vi "MOKE-5-23-22.vi"() -> ()   [LabVIEW 2021]
uses:
  <vilib>/Analysis/NI_AALBase.lvlib
  <vilib>/Analysis/baseanly.llb/Mean (DBL).vi
  <vilib>/Analysis/Matrix/Datatypes/RealMatrix.ctl
  <vilib>/Analysis/Matrix/NI_Matrix.lvlib
panel:
  out "photodiode live avg graph (plots every average, need to update)":cluster{"Y":dbl[], "Y":dbl[]}[](graph)
  out "photodiode final avg graph":cluster{"Y":dbl[], "Y":dbl[]}[](graph)
  out "avgs  (missing last two values but that's ok ig)":dbl[](array[numeric])
  out "avg":dbl
  out "col_arr":dbl[][](array[numeric])
  in  "blank":dbl[](array[numeric])
  out "y_mat":T1
  in  "stop":bool
  in  "Total Loops":dbl
  out "Current Loop":i32
  in  "Time / Step":i64
  in  "Number of Samples":i32=100
  out "Graph For Photodiode":cluster{"Y":dbl[], "Y":dbl[]}[](graph)
  out "Photodiode Level":dbl
  out "Current Voltage":dbl
  in  "Scans From 0 to Max Voltage":i32
  in  "Voltage":dbl
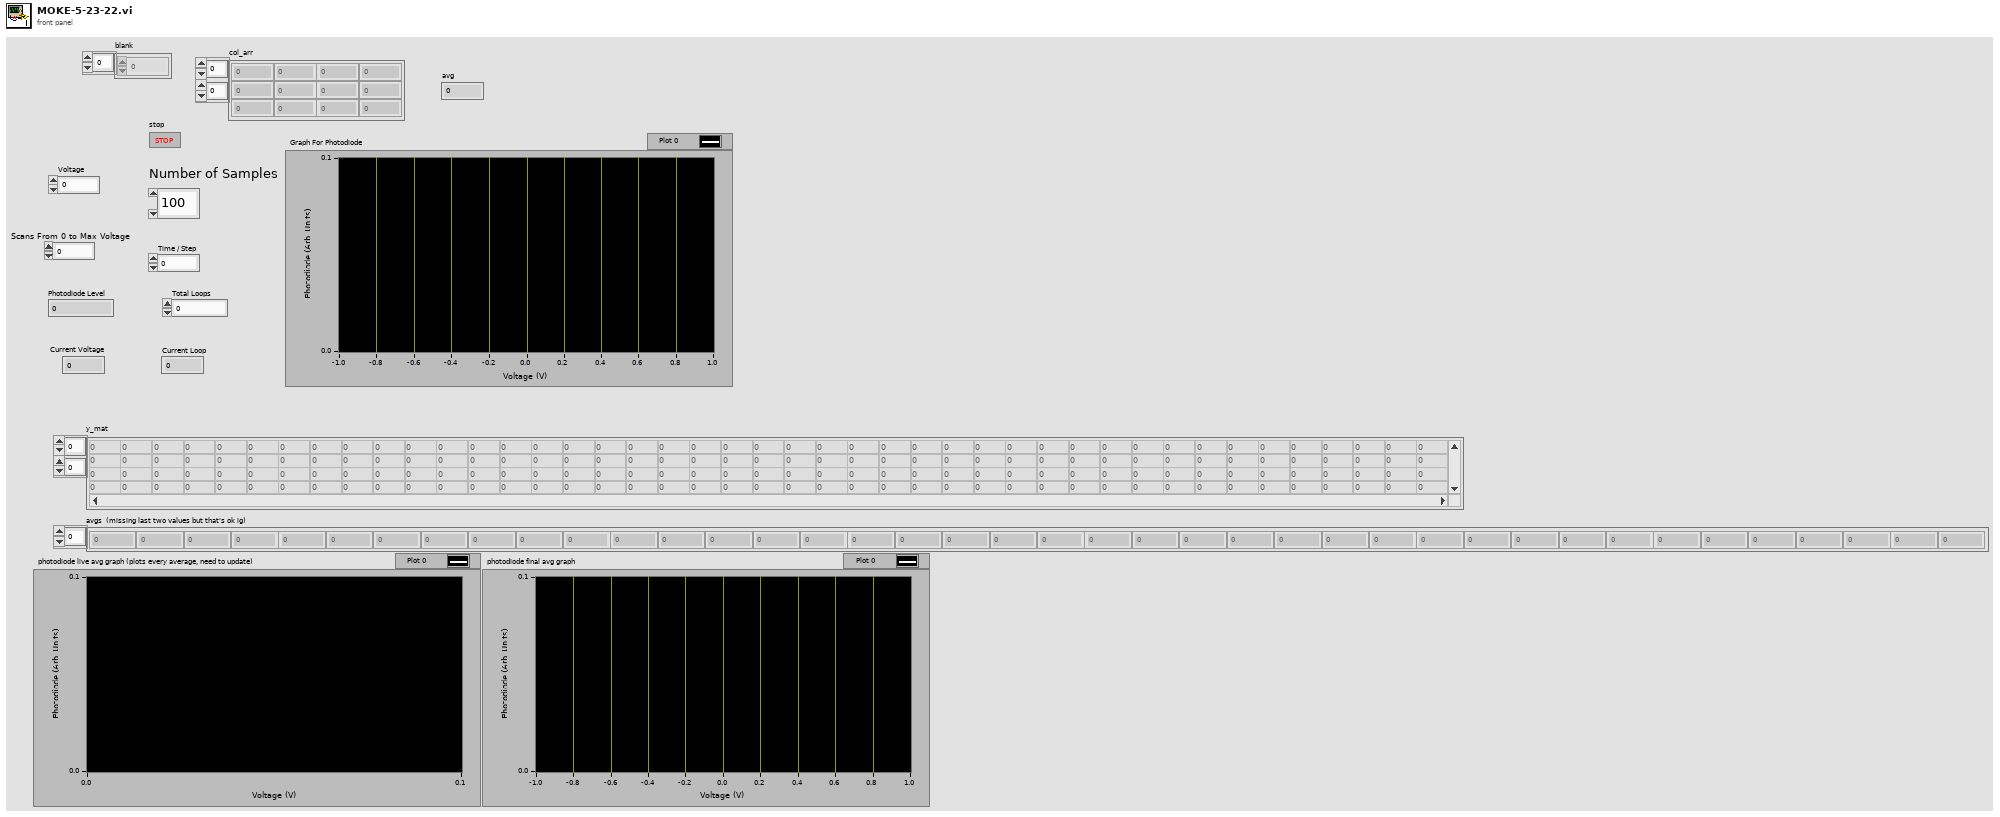
[diagram p1: front panel]
types:
  T1 = typedef "NI_Matrix.lvlib/RealMatrix.ctl" = dbl[][]
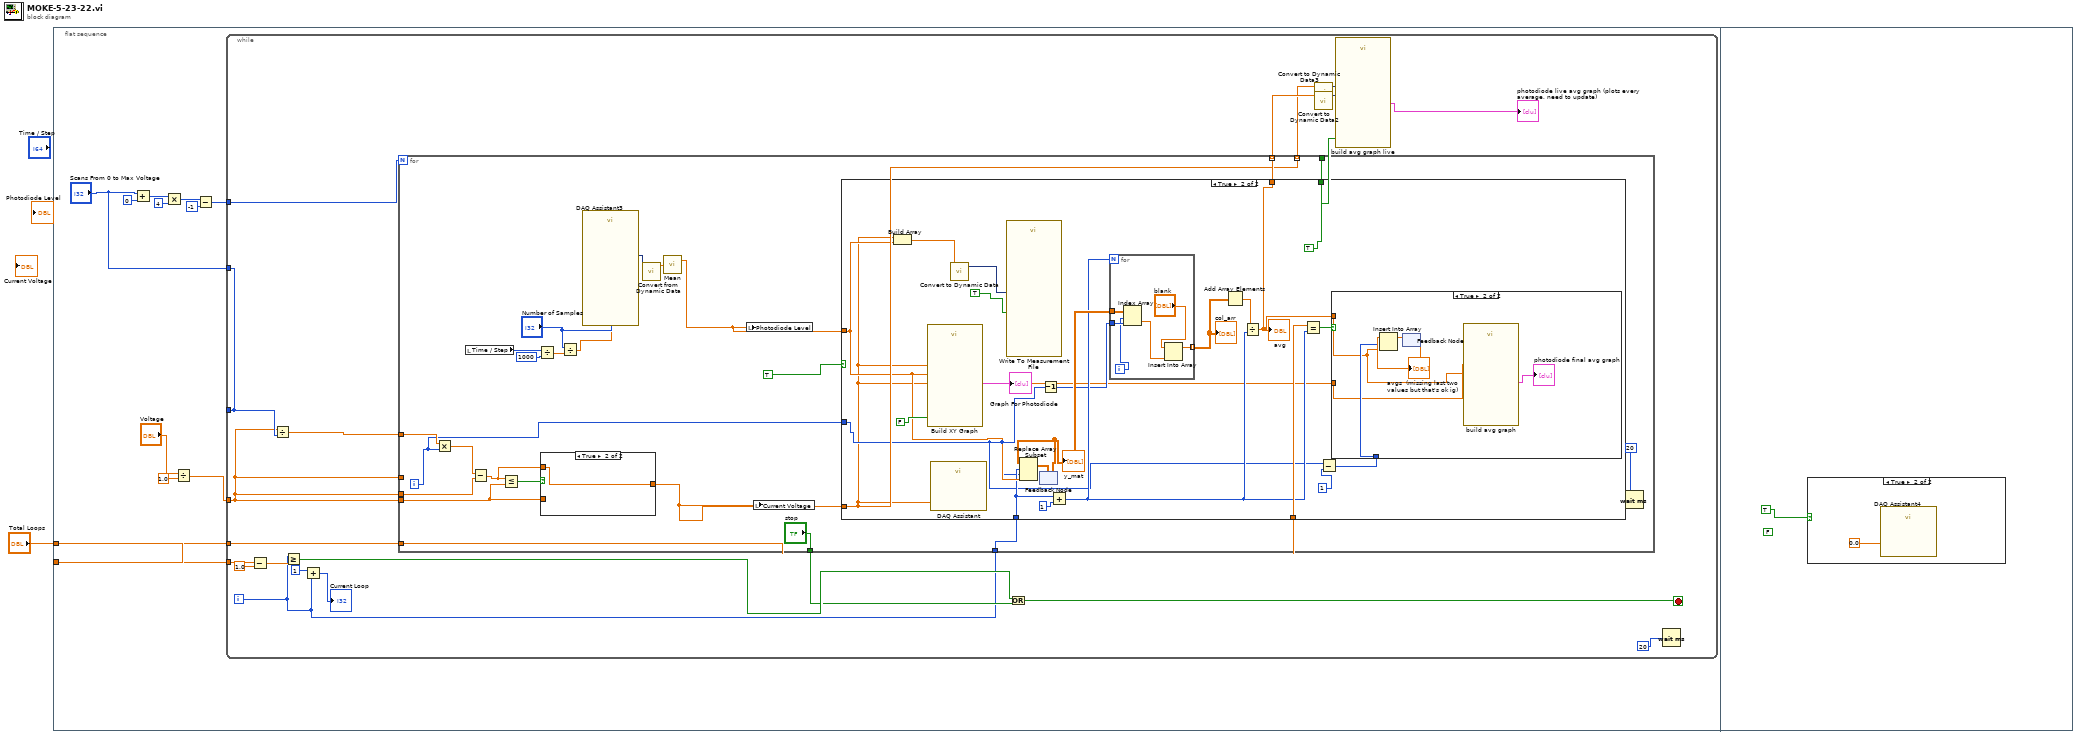
[diagram p0: block diagram]
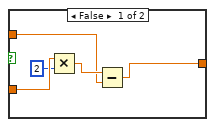
[diagram p2: hidden frame]
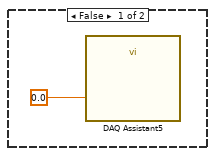
[diagram p5: hidden frame]
diagram:
  n1 = flat-sequence {
    tunnel: "Total Loops" -> [w6]
    tunnel: "Total Loops" -> [w2]
    frame #0 {
      n2 = Add(x="Scans From 0 to Max Voltage", y=0) -> (x+y=w12:i32)
      n3 = Multiply(x=w12, y=4) -> (x*y=w13:i32)
      n4 = Divide(x="Voltage", y=1.0) -> (x/y=w3:dbl)
      n5 = Subtract(x=w13, y=-1) -> (x-y=w8:i32)
      n6 = while {
        tunnel: w6 -> [w33]
        tunnel: [w24] -> _
        tunnel: w8 -> [w25]
        tunnel: "Scans From 0 to Max Voltage" -> [w24]
        tunnel: w3 -> [w23]
        tunnel: w2 -> [w20]
        i -> [w21]
        stop <- w27 stop-if-true
        n7 = Subtract(x=w33, y=1.0) -> (x-y=w32:dbl)
        n8 = Divide(x=w23, y=w24) -> (x/y=w34:dbl)
        n9 = Greater Or Equal?(x=w21, y=w32) -> (x >= y?=w28:bool)
        n10 = Add(x=1, y=w21) -> (x+y=→"Current Loop":i32)
        n11 = for {
          N: w25 -> [_]
          tunnel: w34 -> [w58]
          tunnel: w23 -> [_]
          tunnel: w23 -> [w55]
          tunnel: w23 -> [w51]
          tunnel: ["stop"] -> w26
          tunnel: w21 -> [w39]
          tunnel: w20 -> [w38]
          tunnel: [w37] -> w19
          tunnel: [w36] -> w18 mode=indexing
          tunnel: [w35] -> w17 mode=indexing
          i -> [w40]
          n12 = Multiply(x=w58, y=w40) -> (x*y=w56:dbl)
          n13 = local read "Time / Step"() -> (w47:i64)
          n14 = Subtract(x=w56, y=w55) -> (x-y=w53:dbl)
          n15 = Less Or Equal?(x=w53, y=w51) -> (x <= y?=w54:bool)
          n16 = Divide(x=w47, y=i64 1000) -> (x/y=w48:dbl)
          n17 = case shown="True" w54 {
            tunnel: w53 -> [w60 w64]
            tunnel: [w59 w64] -> w52
            tunnel: w51 -> [w63 _]
            frame False {
              n18 = Multiply(x=w63, y=2) -> (x*y=w61:dbl)
              n19 = Subtract(x=w61, y=w60) -> (x-y=w59:dbl)
            }
            frame True {
            }
          }
          n20 = Divide(x="Number of Samples", y=w48) -> (x/y=w49:dbl)
          n21 = call "DAQ Assistant3"("rate"=w49, "number of samples"="Number of Samples") -> ("data"=w45:dynamicdata)  [unwired: 4 in, 13 out]
          n22 = call "Convert from Dynamic Data"("Dynamic Data Type"=w45) -> ("Array"=w44:dbl[])  [unwired: 3 in]
          n23 = call-poly <vilib>:"Mean.vi"("X"=w44) -> ("mean"=w43:dbl)  [unwired: 1 out]
          n24 = local write "Photodiode Level"(w43) -> ()
          n25 = local write "Current Voltage"(w52) -> ()
          n26 = case shown="True" TRUE {
            tunnel: w52 -> [_ w65]
            tunnel: w43 -> [_ w81]
            tunnel: w40 -> [_ w69]
            tunnel: w39 -> [_ w76]
            tunnel: w38 -> [_ w75]
            tunnel: [_ TRUE] -> w37
            tunnel: [_ w66] -> w36
            tunnel: [_ w65] -> w35
            frame False {
            }
            frame True {
              n27 = Build Array(w65, w81) -> (w84:dbl[])
              n28 = call "Build XY Graph"("Reset"=FALSE, "Y Input"=w81, "X Input"=w65) -> ("XY Graph"=→"Graph For Photodiode":cluster{"X":dbl[], "Y":dbl[]}[])  [unwired: 7 in, 1 out]
              n29 = call "DAQ Assistant"("data"=w65) -> ()  [unwired: 17 in, 2 out]
              n30 = call "Convert to Dynamic Data"("Array"=w84) -> ("Dynamic Data Type"=w82:dynamicdata)  [unwired: 3 in]
              n31 = call "Write To Measurement File"("Signals"=w82, "Enable"=TRUE) -> ()  [unwired: 15 in, 3 out]
              n32 = feedback #1() -> (w79:T1)  [unwired: 1 in]
              "y_mat" <- w79
              n33 = Replace Array Subset(array=w79, new element=w81, index (row)=w76, index (col)=w69) -> (w80:T1)
              n34 = feedback-in #1(w80) -> ()
              n35 = Decrement(x=w69) -> (x-1=w70:i32)
              n36 = Add(x=w76, y=1) -> (x+y=w71:i32)
              n37 = for {
                N: w71 -> [_]
                tunnel: w79 -> [w98]
                tunnel: w70 -> [w94]
                tunnel: [w95] -> w68 mode=indexing
                i -> [w93]
                n38 = Index Array(array=w98, index (row)=w93, index (col)=w94) -> (element=w97:dbl)
                n39 = Insert Into Array(array="blank", new element=w97) -> (w95:dbl[])  [unwired: 1 in]
              }
              "col_arr" <- w68
              n40 = Add Array Elements(numeric array=w68) -> (sum=w78:dbl)
              n41 = Divide(x=w78, y=w71) -> (x/y=w66:dbl)
              "avg" <- w66
              n42 = Equal?(x=w75, y=w71) -> (x = y?=w74:bool)
              n43 = Subtract(x=w69, y=1) -> (x-y=w73:i32)
              n44 = case shown="True" w74 {
                tunnel: w66 -> [_ w88]
                tunnel: w73 -> [_ w90]
                tunnel: w65 -> [_ w89]
                frame False {
                }
                frame True {
                  n45 = feedback #2() -> (w91:dbl[])  [unwired: 1 in]
                  "avgs  (missing last two values but that's ok ig)" <- w91
                  n46 = Insert Into Array(array=w91, index=w90, new element=w88) -> (w92:dbl[])
                  n47 = feedback-in #2(w92) -> ()
                  n48 = call "build avg graph"("Y Input"=w88, "X Input"=w89) -> ("XY Graph"=→"photodiode final avg graph":cluster{"X":dbl[], "Y":dbl[]}[])  [unwired: 8 in, 1 out]
                }
              }
            }
          }
          n49 = Wait (ms)(milliseconds to wait=20) -> ()  [unwired: 1 out]
        }
        n50 = Or(x=w28, y=w26) -> (x .or. y?=w27:bool)
        n51 = call "Convert to Dynamic Data3"("Array"=w17) -> ("Dynamic Data Type"=w14:dynamicdata)  [unwired: 3 in]
        n52 = call "Convert to Dynamic Data2"("Array"=w18) -> ("Dynamic Data Type"=w15:dynamicdata)  [unwired: 3 in]
        n53 = call "build avg graph live"("Reset"=w19, "Y Input"=w15, "X Input"=w14) -> ("XY Graph"=→"photodiode live avg graph (plots every average, need to update)":cluster{"X":dbl[], "Y":dbl[]}[])  [unwired: 7 in, 1 out]
        n54 = Wait (ms)(milliseconds to wait=u32 20) -> ()  [unwired: 1 out]
      }
    }
    frame #1 {
      (unwired) FALSE
      n55 = case shown="True" TRUE {
        frame False {
          n56 = call "DAQ Assistant5"("data"=0.0) -> ()  [unwired: 17 in, 2 out]
        }
        frame True {
          n57 = call "DAQ Assistant4"("data"=0.0) -> ()  [unwired: 17 in, 2 out]
        }
      }
    }
  }
